vi "ZControlSaveData.vi"() -> ()   [LabVIEW 2013]
panel:
  out "Point #":i32
  out "Full file path":path
  out "String":string
  in  "Accept Name":bool
  in  "Base Filename":string
  in  "Voltage":dbl(slide) scale=0.0..10.0 scale format="%.1f"
  out "Temperature = 3V+2":dbl format="%.2f"
  in  "Save Point":bool
  in  "Done":bool
  # "Using CSV Files"
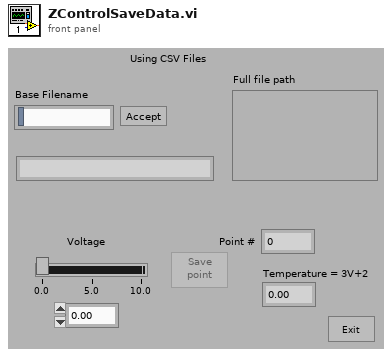
[diagram p1: front panel]
types:
  T1 = enum16{"open", "replace", "create", "open or create", "replace or create", "replace or create with confirmation"}
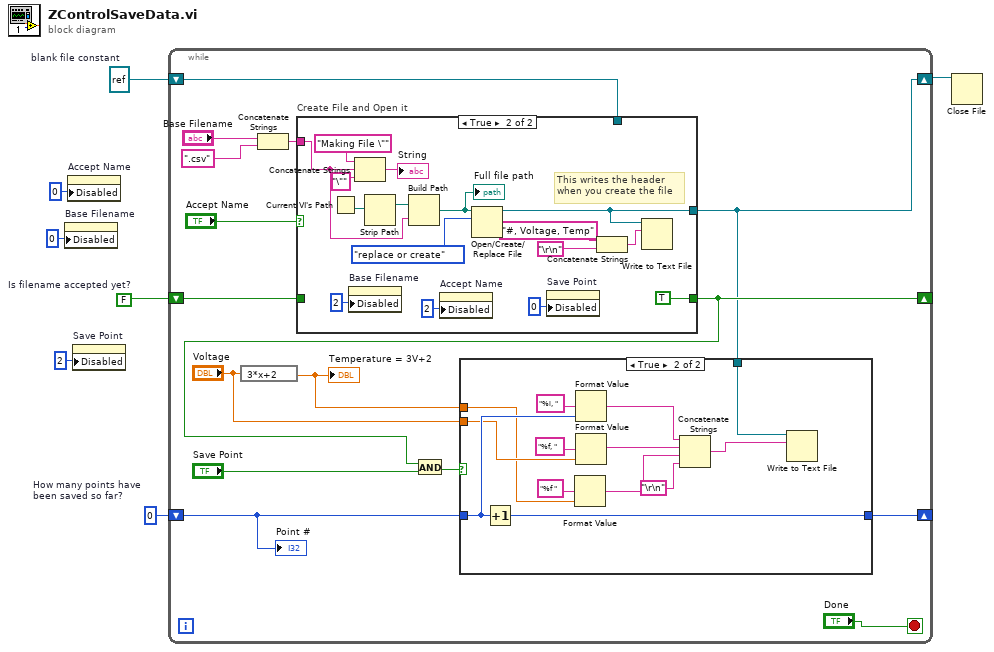
[diagram p0: block diagram]
diagram:
  w2 = refnum<file> refnum  # blank file constant
  w3 = u8 0  # How many points have been saved so far?
  w5 = FALSE  # Is filename accepted yet?
  n1 = property on="Base Filename" class="Str"("Disabled"=u8 0) -> ()  [unwired: 2 in, 2 out]
  n2 = property on="Accept Name" class="Bool"("Disabled"=u8 0) -> ()  [unwired: 2 in, 2 out]
  n3 = property on="Save Point" class="Bool"("Disabled"=u8 2) -> ()  [unwired: 2 in, 2 out]
  n4 = while {
    shift-right: [w14] -> _
    shift-left: w5 -> [w17]
    shift-right: [w11] -> _
    shift-left: w3 -> [w10]
    shift-right: [w9] -> w1
    shift-left: w2 -> [w8]
    stop <- "Done" stop-if-true
    n5 = expression code="3*x+2"("Voltage") -> (w13:dbl)
    "Temperature = 3V+2" <- w13
    n6 = Concatenate Strings("Base Filename", ".csv" ("string")) -> (w18:string)
    n7 = case "Create File and Open it" shown="True" "Accept Name" {
      tunnel: w18 -> [_ w49]
      tunnel: [w37 w39] -> w9
      tunnel: w17 -> [w38 _]
      tunnel: [w38 TRUE ("Is Filename accepted?")] -> w14
      tunnel: w8 -> [w37 _]
      frame False {
      }
      frame True {
        # "This writes the header\nwhen you create the file"
        n8 = Current VI's Path() -> (path=w51:path)
        n9 = property on="Base Filename" class="Str"("Disabled"=u8 2) -> ()  [unwired: 2 in, 2 out]
        n10 = Concatenate Strings("Making File \"" ("string"), w49, "\"" ("string")) -> (→"String":string)
        n11 = Strip Path(path=w51) -> (stripped path=w50:path)  [unwired: 1 out]
        n12 = Build Path(base path=w50, name or relative path=w49) -> (appended path=w48:path)
        "Full file path" <- w48
        n13 = property on="Accept Name" class="Bool"("Disabled"=u8 2) -> ()  [unwired: 2 in, 2 out]
        n14 = Open/Create/Replace File(file path (use dialog)=w48, operation (0:open)=T1."replace or create") -> (refnum out=w39:refnum<file>)  [unwired: 1 in, 5 out]
        n15 = property on="Save Point" class="Bool"("Disabled"=u8 0) -> ()  [unwired: 2 in, 2 out]
        n16 = Concatenate Strings("#, Voltage, Temp" ("string"), "\r\n") -> (w44:string)
        n17 = Write to Text File(file (use dialog)=w39, text=w44) -> ()  [unwired: 2 in, 3 out]
      }
    }
    n18 = And(x=w14, y="Save Point") -> (x .and. y?=w16:bool)
    n19 = case shown="True" w16 {
      tunnel: w13 -> [_ w24]
      tunnel: "Voltage" -> [_ w25]
      tunnel: w10 -> [w23 w30]
      tunnel: [w23 w36] -> w11
      tunnel: w9 -> [_ w34]
      frame False {
      }
      frame True {
        n20 = Increment(x=w30) -> (x+1=w36:u8)
        n21 = Format Value(format string="%f ", value (0)=w24) -> (output string=w28:string)  [unwired: 1 out]
        n22 = Format Value(format string="%i, ", value (0)=w30) -> (output string=w26:string)  [unwired: 1 out]
        n23 = Format Value(format string="%f, ", value (0)=w25) -> (output string=w27:string)  [unwired: 1 out]
        n24 = Concatenate Strings(w26, w27, w28, "\r\n") -> (w35:string)
        n25 = Write to Text File(file (use dialog)=w34, text=w35) -> ()  [unwired: 2 in, 3 out]
      }
    }
    "Point #" <- w10
  }
  n26 = Close File(refnum=w1) -> ()  [unwired: 1 in, 2 out]
